vi "test_rdb_json_decode.vi"() -> (0 "error out":errorcluster, 3 "all_passed":bool)   [LabVIEW 2017]
uses:
  rethinkdb/json/rdb_json_type.ctl
panel:
  out "passed":bool[](array[boolean])
  out "values":T1(array[cluster])
  in  "test_cases":T3(array[cluster])
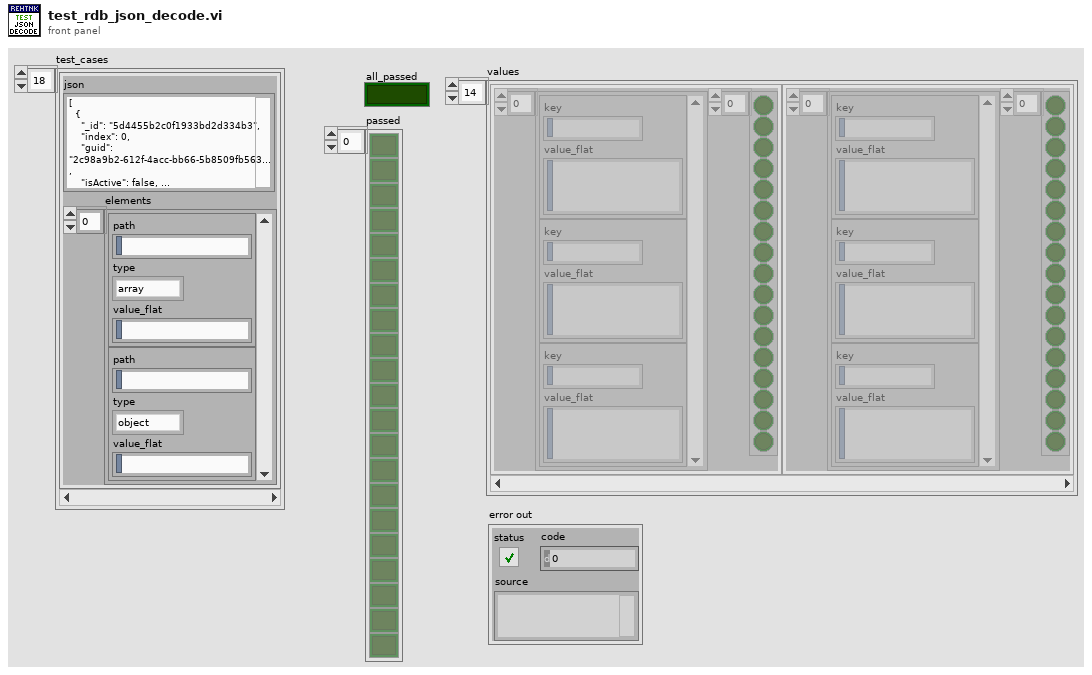
[diagram p1: front panel]
types:
  T1 = cluster{cluster{"key":string, "value_flat":string}[], bool[]}[]
  T2 = typedef "rdb_json_type.ctl" = enum8{"null", "bool", "int", "uint", "float", "string", "array", "object", "invalid"}
  T3 = cluster{"json":string, "elements":cluster{"path":string, "type":T2, "value_flat":string}[]}[]
  T4 = cluster{"path":string, "type":T2, "value_flat":string}[]
  T5 = typedef "rdb_json_element.ctl" = cluster{"key":string, "type":T2, "indent":i32, "start":i32, "vstart":i32, "end":i32, "value":variant}
  T6 = cluster{"path":string, "type":T2, "value_flat":string}
  T7 = cluster{cluster{"key":string, "value_flat":string}[], bool[]}
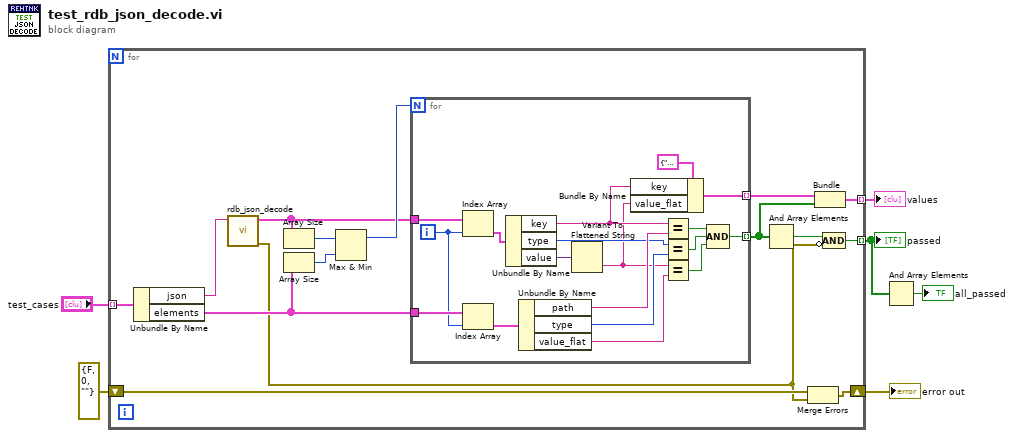
[diagram p0: block diagram]
diagram:
  n1 = for {
    tunnel: "test_cases" -> [w21] mode=indexing
    tunnel: [w15] -> w5 mode=indexing
    tunnel: [w12] -> w4 mode=indexing
    shift-right: [w11] -> w1
    shift-left: errorcluster {"status"=FALSE, "code"=0, "source"=""} ("error out") -> [w10]
    n2 = Unbundle By Name(w21) -> ("json"=w8:string, "elements"=w20:T4)
    n3 = call "rdb_json_decode.vi"("json"=w8) -> ("error out"=w9:errorcluster, "elements"=w7:T5[])  [unwired: 9 in]
    n4 = Array Size(array=w7) -> (size(s)=w19:i32)
    n5 = Array Size(array=w20) -> (size(s)=w18:i32)
    n6 = Max & Min(x=w19, y=w18) -> (max(x,y)=w17:i32)  [unwired: 1 out]
    n7 = for {
      N: w17 -> [_]
      tunnel: w7 -> [w39]
      tunnel: w20 -> [w38]
      tunnel: [w31] -> w16 mode=indexing
      tunnel: [w27] -> w14 mode=indexing
      i -> [w37]
      n8 = Index Array(array=w39, index=w37) -> (element=w36:T5)
      n9 = Index Array(array=w38, index=w37) -> (element=w35:T6)
      n10 = Unbundle By Name(w36) -> ("key"=w24:string, "type"=w23:T2, "value"=w34:variant)
      n11 = Unbundle By Name(w35) -> ("path"=w33:string, "type"=w26:T2, "value_flat"=w30:string)
      n12 = Variant To Flattened String(Variant=w34) -> (data string=w22:string)  [unwired: 1 out]
      n13 = Bundle By Name(cluster=cluster{"key":string, "value_flat":string} {"key"="", "value_flat"=""} ("element"), "key"=w24, "value_flat"=w22) -> (w31:cluster{"key":string, "value_flat":string})
      n14 = Equal?(x=w24, y=w33) -> (x = y?=w28:bool)
      n15 = Equal?(x=w23, y=w26) -> (x = y?=w25:bool)
      n16 = Equal?(x=w22, y=w30) -> (x = y?=w29:bool)
      n17 = Compound Arithmetic op=AND(w28, w25, w29) -> (w27:bool)
    }
    n18 = And Array Elements(Boolean array=w14) -> (logical AND=w13:bool)
    n19 = Merge Errors(w10, w9) -> (w11:errorcluster)
    n20 = Bundle(w16, w14) -> (w15:T7)  [unwired: 1 in]
    n21 = Compound Arithmetic op=AND(w13, invert w9) -> (w12:bool)
  }
  "values" <- w5
  "passed" <- w4
  "error out" <- w1
  n22 = And Array Elements(Boolean array=w4) -> (logical AND=→"all_passed":bool)
